vi "VISA_Read_1CH.vi"() -> ()   [LabVIEW 2019]
uses:
  <vilib>/Instr/_visa.llb/VISA Configure Serial Port (Instr).vi
  <vilib>/Utility/file.llb/Write Delimited Spreadsheet (DBL).vi
panel:
  out "Status Serial":errorcluster
  in  "Stop and Save Read":bool
  in  "Start Read":bool
  in  "baud rate (9600)":u32=115200
  in  "data bits (8)":u8=8 min=5 max=8 step=1
  in  "VISA resource name":refnum<visa-resource-name>
  out "Buffer Array":dbl[](array[numeric])
  out "Read Buffer":string
  out "Status Read":errorcluster
  out "Buffer Plot":dbl[](graph)
  # "Conversão Para Inteiro"
  # "Controle da porta Serial USB"
  # "Controle da Leitura"
  # "Resultado da Leitura"
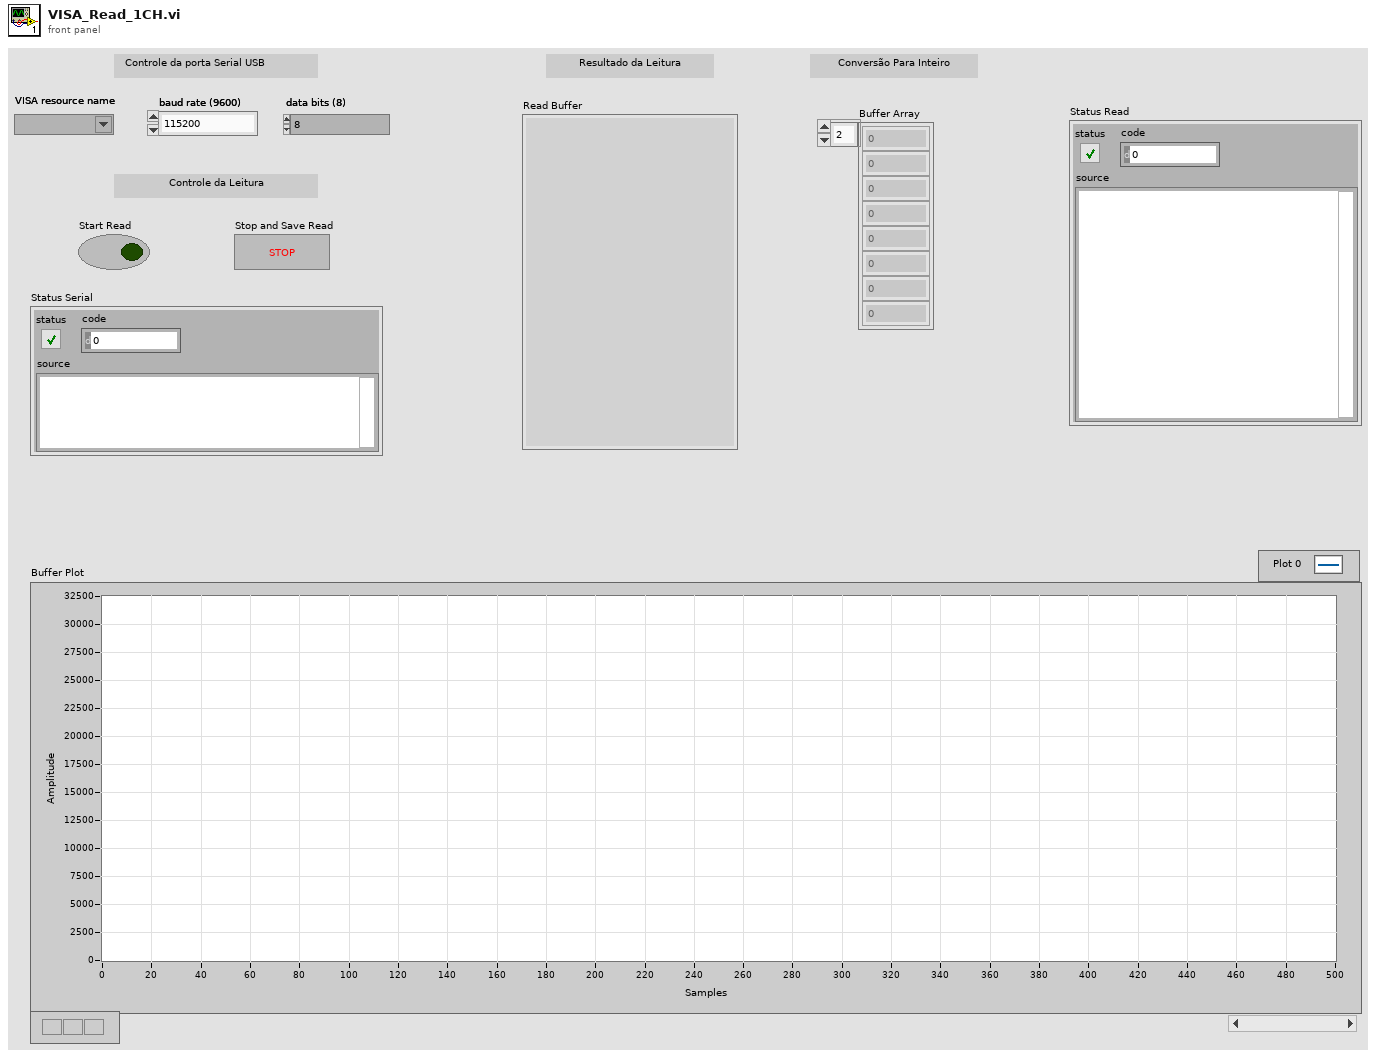
[diagram p1: front panel]
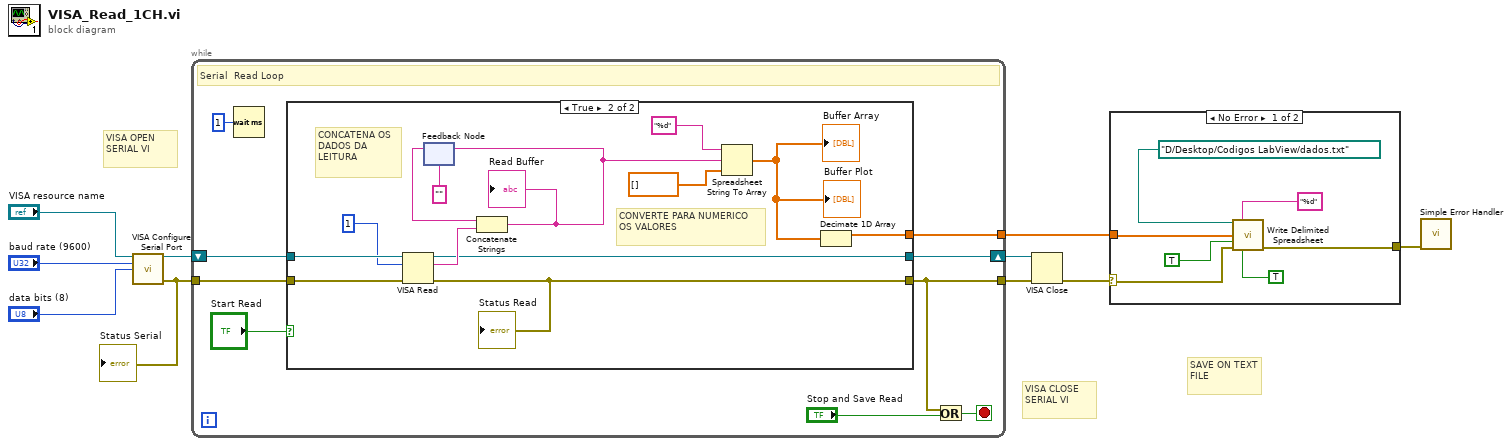
[diagram p0: block diagram]
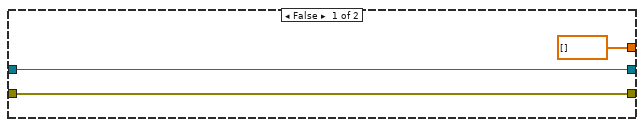
[diagram p3: hidden frame]
diagram:
  # "SAVE ON TEXT FILE"
  # "VISA CLOSE SERIAL VI"
  # "VISA OPEN SERIAL VI"
  n1 = call-poly "VISA Configure Serial Port"("VISA resource name"="VISA resource name", "baud rate (9600)"="baud rate (9600)", "data bits (8)"="data bits (8)") -> ("VISA resource name out"=w9:refnum<visa-resource-name>, "error out"=w7:errorcluster)  [unwired: 11 in]
  "Status Serial" <- w7
  n2 = while {
    tunnel: w7 -> [w19]
    tunnel: [w17] -> w10
    shift-right: [w14] -> w8
    shift-left: w9 -> [w15]
    tunnel: [w11] -> w2
    stop <- w18 stop-if-true
    # "Serial  Read Loop"
    n3 = Wait (ms)(milliseconds to wait=u32 1) -> ()  [unwired: 1 out]
    n4 = case shown="True" "Start Read" {
      tunnel: w19 -> [w21 w35]
      tunnel: [w21 w34] -> w17
      tunnel: w15 -> [w22 w30]
      tunnel: [w22 w29] -> w14
      tunnel: [dbl[] [] w23] -> w11
      frame False {
      }
      frame True {
        # "CONVERTE PARA NUMERICO OS VALORES"
        # "CONCATENA OS DADOS DA LEITURA"
        n5 = VISA Read(VISA resource name=w30, byte count=u32 1, error in (no error)=w35) -> (VISA resource name out=w29:refnum<visa-resource-name>, read buffer=w33:string, error out=w34:errorcluster)  [unwired: 1 out]
        "Status Read" <- w34
        n6 = feedback #1("") -> (w32:string)
        n7 = Concatenate Strings(w32, w33) -> (w28:string)
        "Read Buffer" <- w28
        n8 = feedback-in #1(w28) -> ()
        n9 = Spreadsheet String To Array(format string="%d", spreadsheet string=w28, array type (2D Dbl)=dbl[] []) -> (array=w24:dbl[])  [unwired: 1 in]
        "Buffer Array" <- w24
        "Buffer Plot" <- w24
        n10 = Decimate 1D Array(w24) -> (w23:dbl[])  [unwired: 1 out]
      }
    }
    n11 = Or(x=w17, y="Stop and Save Read") -> (x .or. y?=w18:bool)
  }
  n12 = VISA Close(VISA resource name=w8, error in (no error)=w10) -> (error out=w3:errorcluster)
  n13 = case shown="No Error" w3 {
    selector: w3 -> [w37 w43]
    tunnel: w2 -> [w36 _]
    tunnel: [w38 w43] -> w1
    frame No Error {
      n14 = call-poly <vilib>:"Write Delimited Spreadsheet.vi"("file path (dialog if empty)"=path "D:/Desktop/Codigos LabView/dados.txt", "format (%.3f)"="%d", "1D data"=w36, "append to file? (new file:F)"=TRUE, "error in (no error)"=w37, "transpose? (no:F)"=TRUE) -> ("error out"=w38:errorcluster)  [unwired: 8 in, 1 out]
    }
    frame Error {
    }
  }
  n15 = call <vilib>:"Simple Error Handler.vi"("error in (no error)"=w1) -> ()  [unwired: 4 in, 5 out]
